vi "AMC e.bloxx Read Value - CORE.vi"(8 "error in (no error)":errorcluster, 9 "Channel":i32, 10 "Module Address":i32, 11 "VISA Resource Name":refnum<visa-resource-name>) -> (0 "error out":errorcluster, 2 "Value":dbl, 3 "VISA Resource Name out":refnum<visa-resource-name>)   [LabVIEW 2013]
doc: "<B>AMC - Analytik & Messtechnik GmbH Chemnitz</B>\n\nLabVIEW Drivers for e.bloxx series from Gantner Instruments\n\nThis VI is a driver subroutine and should not be used in an application. It reads a value from a variable specified by <B>Module Address</B> and <B>Variable</B> (starts counting with 0)."
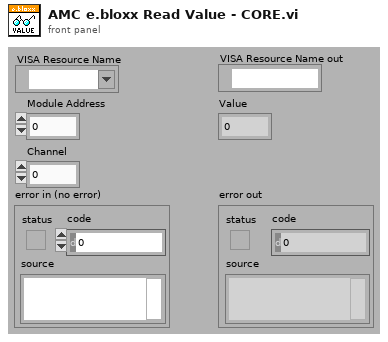
[diagram p1: front panel]
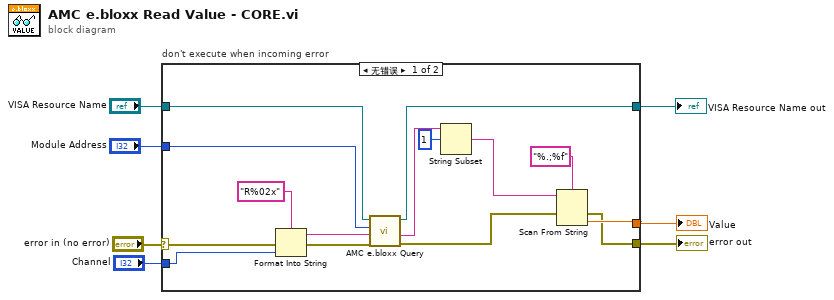
[diagram p0: block diagram]
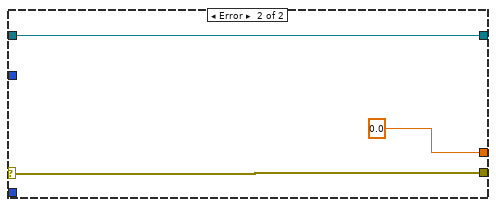
[diagram p2: hidden frame]
diagram:
  n1 = case "don't execute when incoming error" shown="无错误" "error in (no error)" {
    selector: "error in (no error)" -> [w15 w25]
    tunnel: [w12 w25] -> w6
    tunnel: "VISA Resource Name" -> [w21 w24]
    tunnel: "Module Address" -> [w22 _]
    tunnel: [w20 w24] -> w3
    tunnel: "Channel" -> [w13 _]
    tunnel: [w18 0.0] -> w1
    frame No Error {
      n2 = Format Into String(format string="R%02x", error in=w15, w13) -> (resulting string=w11:string, error out=w14:errorcluster)  [unwired: 1 in]
      n3 = call "AMC e.bloxx Query.vi"("error in (no error)"=w14, "Module Command"=w11, "Module Address"=w22, "VISA Resource Name"=w21) -> ("error out"=w9:errorcluster, "Module Response"=w17:string, "VISA Resource Name out"=w20:refnum<visa-resource-name>)  [unwired: 5 in]
      n4 = String Subset(string=w17, offset (0)=1) -> (substring=w8:string)  [unwired: 1 in]
      n5 = Scan From String(format string="%.;%f", input string=w8, error in=w9) -> (error out=w12:errorcluster, output 1=w18:dbl)  [unwired: 2 in, 2 out]
    }
    frame Error {
    }
  }
  "error out" <- w6
  "VISA Resource Name out" <- w3
  "Value" <- w1
